vi "Division.vi"(8 "error in (no error)":errorcluster, 11 "Calculadora in":refnum<class "Calculadora.lvclass">) -> (0 "error out":errorcluster, 3 "Calculadora out":refnum<class "Calculadora.lvclass">)   [LabVIEW 2020, in "Calculadora.lvlib" / "Calculadora.lvclass"]
uses:
  Calculadora.lvclass
  Calculadora.lvclass/Calculadora.ctl
  <vilib>/ActorFramework/Actor/Actor.lvclass
  Calculadora Messages/Display Resultado Msg/Display Resultado Msg.lvclass
  C:/Program Files (x86)/National Instruments/LabVIEW 2020/vi.lib/ActorFramework/Actor/Actor.lvclass
  D:/Storage/Source Code/Clase AF/ClaseAF/02 QMH/Calculadora/Calculadora/Calculadora.lvclass
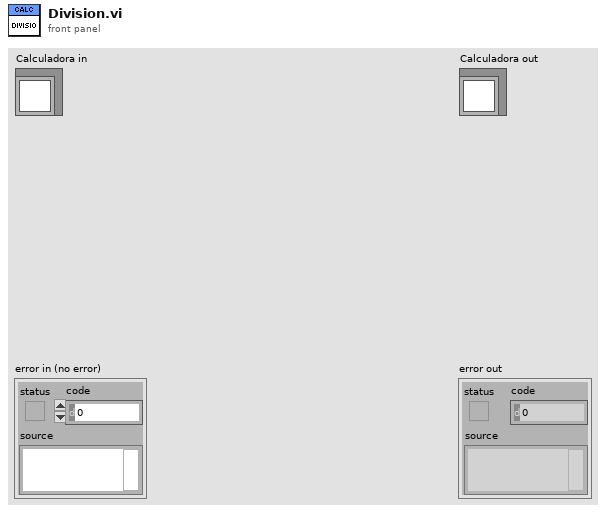
[diagram p1: front panel]
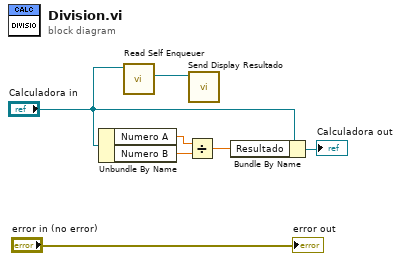
[diagram p0: block diagram]
diagram:
  n1 = Unbundle By Name("Calculadora in") -> ("Numero A"=w5:dbl, "Numero B"=w4:dbl)
  n2 = call <vilib>:"Read Self Enqueuer.vi"("Actor"="Calculadora in") -> ("Self Enqueuer"=w1:refnum<class "Message Enqueuer.lvclass">)  [unwired: 10 in]
  n3 = Divide(x=w5, y=w4) -> (x/y=w3:dbl)
  n4 = call "Send Display Resultado.vi"("Message Enqueuer"=w1) -> ()  [unwired: 9 in, 2 out]
  n5 = Bundle By Name(cluster="Calculadora in", "Resultado"=w3) -> (→"Calculadora out":refnum<class "Calculadora.lvclass">)
  "error out" <- "error in (no error)"
